vi "Untitled 2.vi"() -> ()   [LabVIEW 2020]
uses:
  Control/State - Query Type.ctl
panel:
  out "Query String":string="SELECT `config_name`,`value` FROM `configuration` ORDER BY `id` ASC "
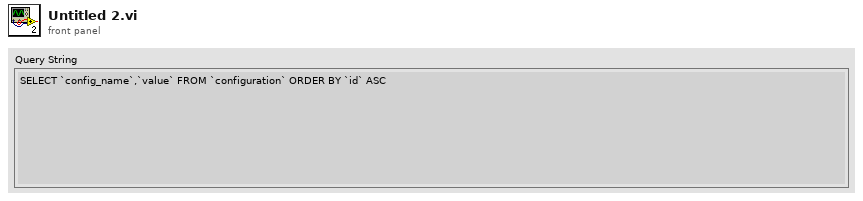
[diagram p1: front panel]
types:
  T1 = typedef "State - Query Type.ctl" = enum16{"SELECT", "UPDATE", "INSERT INTO", "TRUNCATE TABLE"}
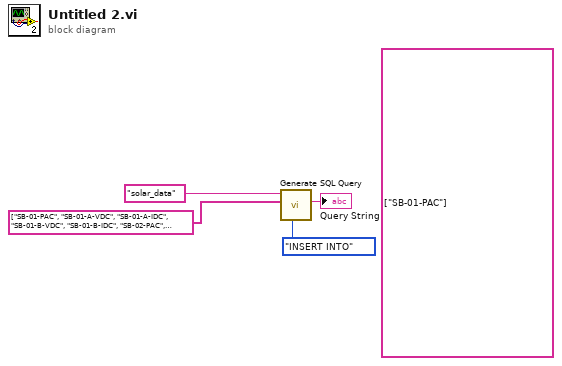
[diagram p0: block diagram]
diagram:
  (unwired) string[] ["SB-01-PAC"] ("Values")
  n1 = call "Generate SQL Query.vi"("Query type"=State_-_Query_Type."INSERT INTO", "Column Name"=string[] ["SB-01-PAC", "SB-01-A-VDC", "SB-01-A-IDC", "SB-01-B-VDC", "SB-01-B-IDC", "SB-02-PAC", "SB-02-A-VDC", "SB-02-A-IDC", "SB-02-B-VDC", "SB-02-B-IDC", "BANK-01-SOC", "BANK-01-VBAT", "BANK-01-IBAT", "BANK-01-TBAT", "BANK-02-SOC", "BANK-02-VBAT", "BANK-02-IBAT", "BANK-02-TBAT", "SI-M-PAC", "SI-M-L1", "SI-M-L2", "SI-M-L3", "SI-M-FREQ", "SI-01-PAC", "SI-01-L1", "SI-01-L2", "SI-01-L3", "SI-01-FREQ", "PM-01-PAC", "PM-01-VAC", "PM-01-IAC", "PM-01-FREQ"] ("array w/ subset deleted"), "Table Name"="solar_data") -> ("Query String"=→"Query String":string)  [unwired: 7 in, 1 out]
